vi "Simulation - Tank Level RT SO sim.vi"() -> ()   [LabVIEW 2025]
doc: "This example demonstrates a process simulation for a tank level. The process has added noise, valve deadband, lag, and deadtime. A level controller adjusts the inflow to a tank. An on/off valve serves as a drain that you can click on to operate. This s-valve represents a change in the process loading. You also can switch this VI from automatic control to manual control."
uses:
  <vilib>/addons/control/pid/NI_PID_pid.lvlib
  <vilib>/addons/control/pid/pid.llb/PID Advanced (DBL).vi
  home/lvuser/natinst/tank3_lvrt.so
  Process.ctl
panel:
  in  "stop":bool
  in  "process":T1
  in  "Tab Control":enum32{"Introduction", "Operation"}(tab)=enum."Operation"
  out "flow_out":dbl=35.0
  out "Flow sensor":bool=TRUE
  in  "HV-101":bool=TRUE
  out "tank level":dbl(slide)=38.064516129032256 scale=0.0..100.0 scale format="%#.2g"
  out "Valve":bool=TRUE
  in  "LCV-101":dbl(knob)=34.81999593540954 scale=0.0..100.0
  in  "Auto":bool=TRUE
  out "Process Chart":T2(graph)={"initial PV"=71.76166045878605, "SP(%)"=71.24183006535948, "output"=34.81999593540954}
  in  "Setpoint":dbl(slide)=26.797385620915033 scale=0.0..100.0
  in  "PID parameters (LIC 101)":T3={"Kc"=10.0, "Ti (min)"=0.05, "Td (min)"=0.0001} {"Td (min)" format="%#.6f"; "Ti (min)" format="%#.4f"; "Kc" format="%#.4f"}
  out "flow_in":dbl=34.81999593540954
  # "Tank Level Control"
  # "Overview: This example demonstrates a process simulation for a tank level.  The process has added noise, valve deadband, lag, and deadtime.  A level controller adjusts the inflow to a tank.  An on/off valve serves as a drain that you can click on to operate.  This s-valve represents a change in the process loading.  You also can switch this VI from automatic control to manual control.\nInstructions:\n1. Run the VI.\n2. Verify the PID controller in closed-loop to track the setpoint.\n3. Change the setpoint to another value and verify the controller tracking the new setpoint.\n4. Apply a disturbance to the system by switching the valve HV 102 (click on the valve symbol). You will see the controller recovering fro the change.\n5. Change PID gains and see if you can improve its performance without going unstable.\n6. Switch to manual mode and see if you can control the level by changing the Valve LVC 101.\n7. Click Stop to stop the VI."
  # "ISA Symbology: The diagram uses the ISA Symbology used for control"
  # "Loop 101"
  # "Level Controller at the control room"
  # "Level Transmitter on the field"
  # "Level Control Valve on the field"
  # "Hand Control Valve on the field"
  # "HV"
  # "102"
  # "LCV"
  # "101"
  # "LIC"
  # "101"
  # "LT"
  # "101"
  # "Slow Leak"
  # "Click to operate"
  # "HV"
  # "102"
  # "LCV"
  # "101"
  # "LIC"
  # "101"
  # "LT"
  # "101"
  # "Manual"
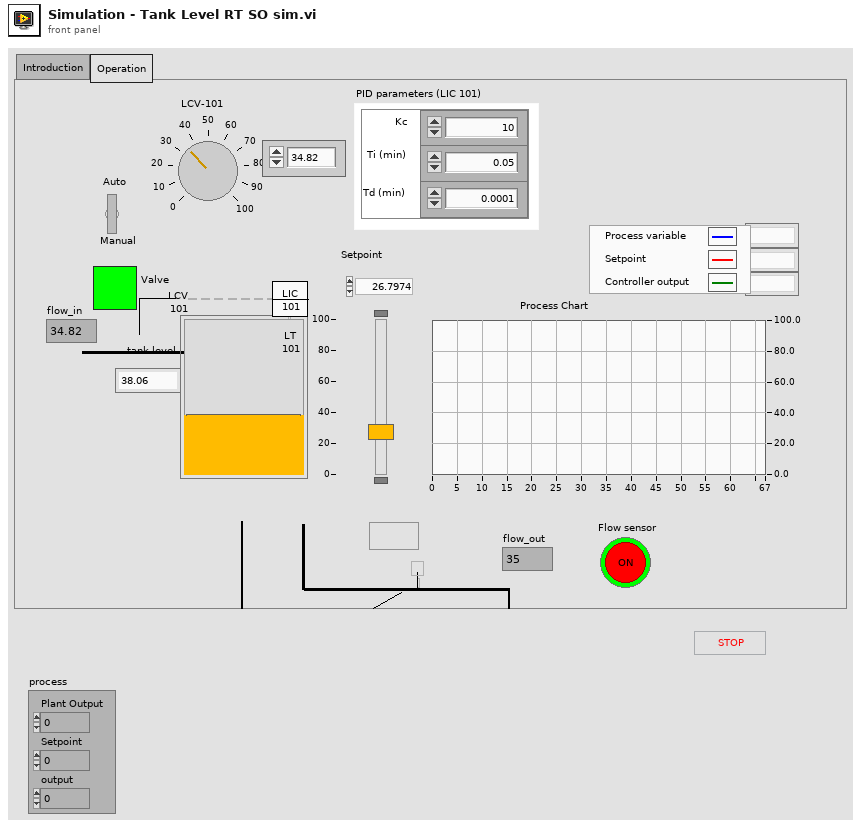
[diagram p1: front panel]
types:
  T1 = typedef "Process.ctl" = cluster{"Plant Output":dbl, "Setpoint":dbl, "output":dbl}
  T2 = cluster{"initial PV":dbl, "SP(%)":dbl, "output":dbl}
  T3 = cluster{"Kc":dbl, "Ti (min)":dbl, "Td (min)":dbl}
  T4 = cluster{"static gain":dbl, "lag (s)":dbl, "deadtime (s)":dbl, "load":dbl, "deadband":dbl, "sensor noise":dbl, "initial PV":dbl, "plant noise":dbl}
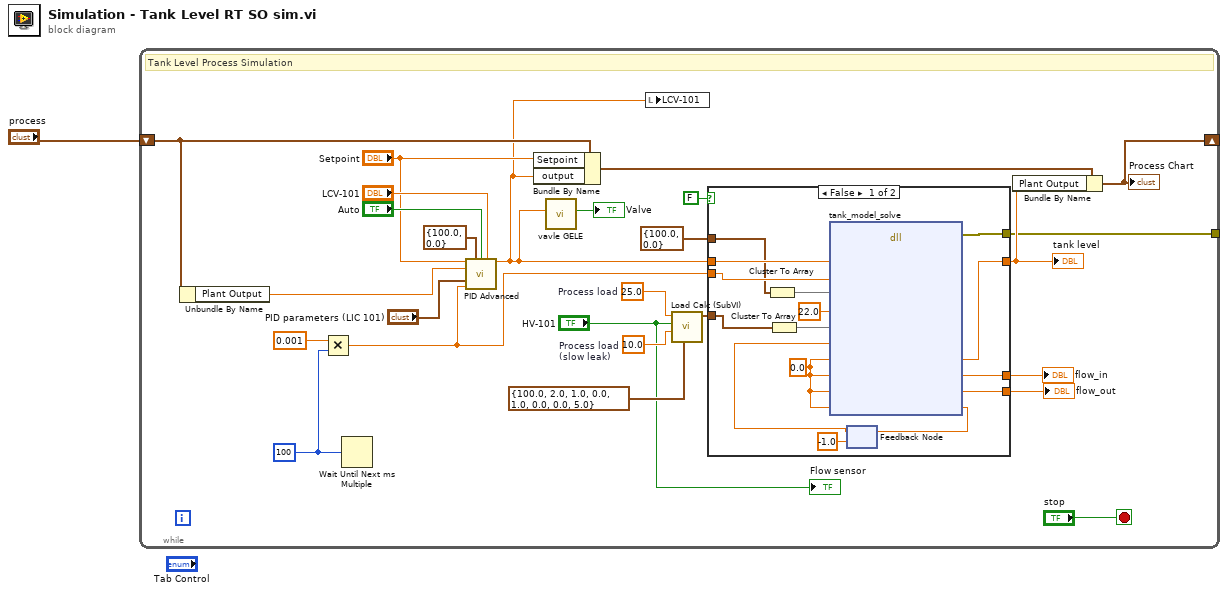
[diagram p0: block diagram]
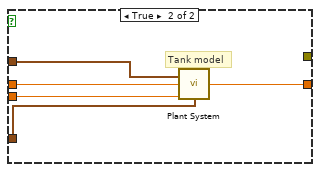
[diagram p2: hidden frame]
diagram:
  n1 = while {
    shift-right: [w10] -> _
    shift-left: "process" -> [w9]
    tunnel: [w5] -> _
    stop <- "stop" stop-if-true
    w21 = u32 100
    w15 = 25.0  # Process load
    w12 = 10.0  # Process load (slow leak)
    # "Tank Level Process Simulation"
    n2 = Unbundle By Name(w9) -> ("Plant Output"=w8:dbl)
    n3 = Multiply(x=0.001, y=w21) -> (x*y=w20:dbl)
    n4 = Wait Until Next ms Multiple(millisecond multiple=w21) -> ()  [unwired: 1 out]
    n5 = call-poly <vilib>:"PID Advanced.vi"("setpoint"="Setpoint", "output range"=cluster{"output high":dbl, "output low":dbl} {"output high"=100.0, "output low"=0.0}, "auto? (T)"="Auto", "manual control"="LCV-101", "process variable"=w8, "PID gains"="PID parameters (LIC 101)", "dt (s)"=w20) -> ("output"=w7:dbl)  [unwired: 7 in, 1 out]
    n6 = Bundle By Name(cluster=w9, "Setpoint"="Setpoint", "output"=w7) -> (w16:T1)
    n7 = call "vavle GELE.vi"("output"=w7) -> ("T=Opening"=→"Valve":bool)  [unwired: 10 in]
    n8 = local write "LCV-101"(w7) -> ()
    n9 = call "Load Calc (SubVI).vi"("process parameters in"=T4 {"static gain"=100.0, "lag (s)"=2.0, "deadtime (s)"=1.0, "load"=0.0, "deadband"=1.0, "sensor noise"=0.0, "initial PV"=0.0, "plant noise"=5.0} ("process parameters"), "Leak load"=w12, "HV-101"="HV-101", "Process load"=w15) -> ("process parameters out"=w14:T4)  [unwired: 7 in]
    n10 = case shown="False" FALSE {
      tunnel: cluster{"output high":dbl, "output low":dbl} {"output high"=100.0, "output low"=0.0} ("output saturation range") -> [w40 w47]
      tunnel: w20 -> [w41 w46]
      tunnel: [w32 w45] -> w19
      tunnel: w14 -> [w37 w44]
      tunnel: w7 -> [w42 w43]
      tunnel: [w31 _] -> w5
      tunnel: [w29 _] -> w4
      tunnel: [w28 _] -> w3
      frame False {
        w33 = 0.0 ("initial_level")
        n11 = Cluster To Array(cluster=w40) -> (array=w39:dbl[])
        n12 = Cluster To Array(cluster=w37) -> (array=w36:dbl[])
        n13 = feedback #1(-1.0 ("state_out")) -> (w34:dbl)
        n14 = dll-call lib="home/lvuser/natinst/tank3_lvrt.so" fn="tank_model_solve"("Valve_pos"=w42, "dt"=w41, "range_vals"=w39, "initial_level"=22.0, "process_params"=w36, "state_in"=w34, "measured_level"=w33, "flow_in"=w33, "flow_out"=w33, "state_out"=w33) -> (error out=w31:errorcluster, "measured_level"=w32:dbl, "flow_in"=w29:dbl, "flow_out"=w28:dbl, "state_out"=w35:dbl)  [unwired: 10 in, 1 out]
        n15 = feedback-in #1(w35) -> ()
      }
      frame True {
        # "Tank model"
        n16 = call "Plant System.vi"("output saturation range"=w47, "Plant Input"=w43, "dt (s)"=w46, "process parameters"=w44) -> ("Plant Output"=w45:dbl)  [unwired: 11 in]
      }
    }
    "tank level" <- w19
    "flow_in" <- w4
    "flow_out" <- w3
    n17 = Bundle By Name(cluster=w16, "Plant Output"=w19) -> (w10:T1)
    "Process Chart" <- w10
    "Flow sensor" <- "HV-101"
  }
